vi "Strip apostrophe.vi"   [LabVIEW 2014, in "_lvcicd_support_2014.lvlib"]
uses:
  _lvcicd_support_2014.lvlib
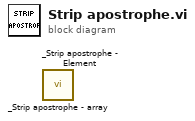
[diagram p0: block diagram]
diagram:
  n1 = call "_Strip apostrophe - array.vi"() -> ()  [unwired: 11 in, 1 out]
  n2 = call "_Strip apostrophe - Element.vi"() -> ()  [unwired: 11 in, 1 out]
